vi "main.vi"() -> ()   [LabVIEW 2013, in "Octoplus_LIDAR.lvlib"]
uses:
  <userlib>/Octoplus_LIDAR/Octoplus_LIDAR.lvlib
  <vilib>/Analysis/NI_AALBase.lvlib
panel:
  in  "Nbr of lines in Image":u32=600
  in  "File Path":path=path "D:/Sat25"
  in  "Capture":bool
  in  "Record data":bool
  in  "Timeslot (cw, ts1, ts2)":i32(knob)=1 scale=0.0..2.0
  out "Background":dbl[](graph)
  in  "start":bool
  out "Signal":dbl[][](graph)
  out "iteration":i32
  in  "stop":bool
  in  "error in (no error)":errorcluster
  out "error out":errorcluster
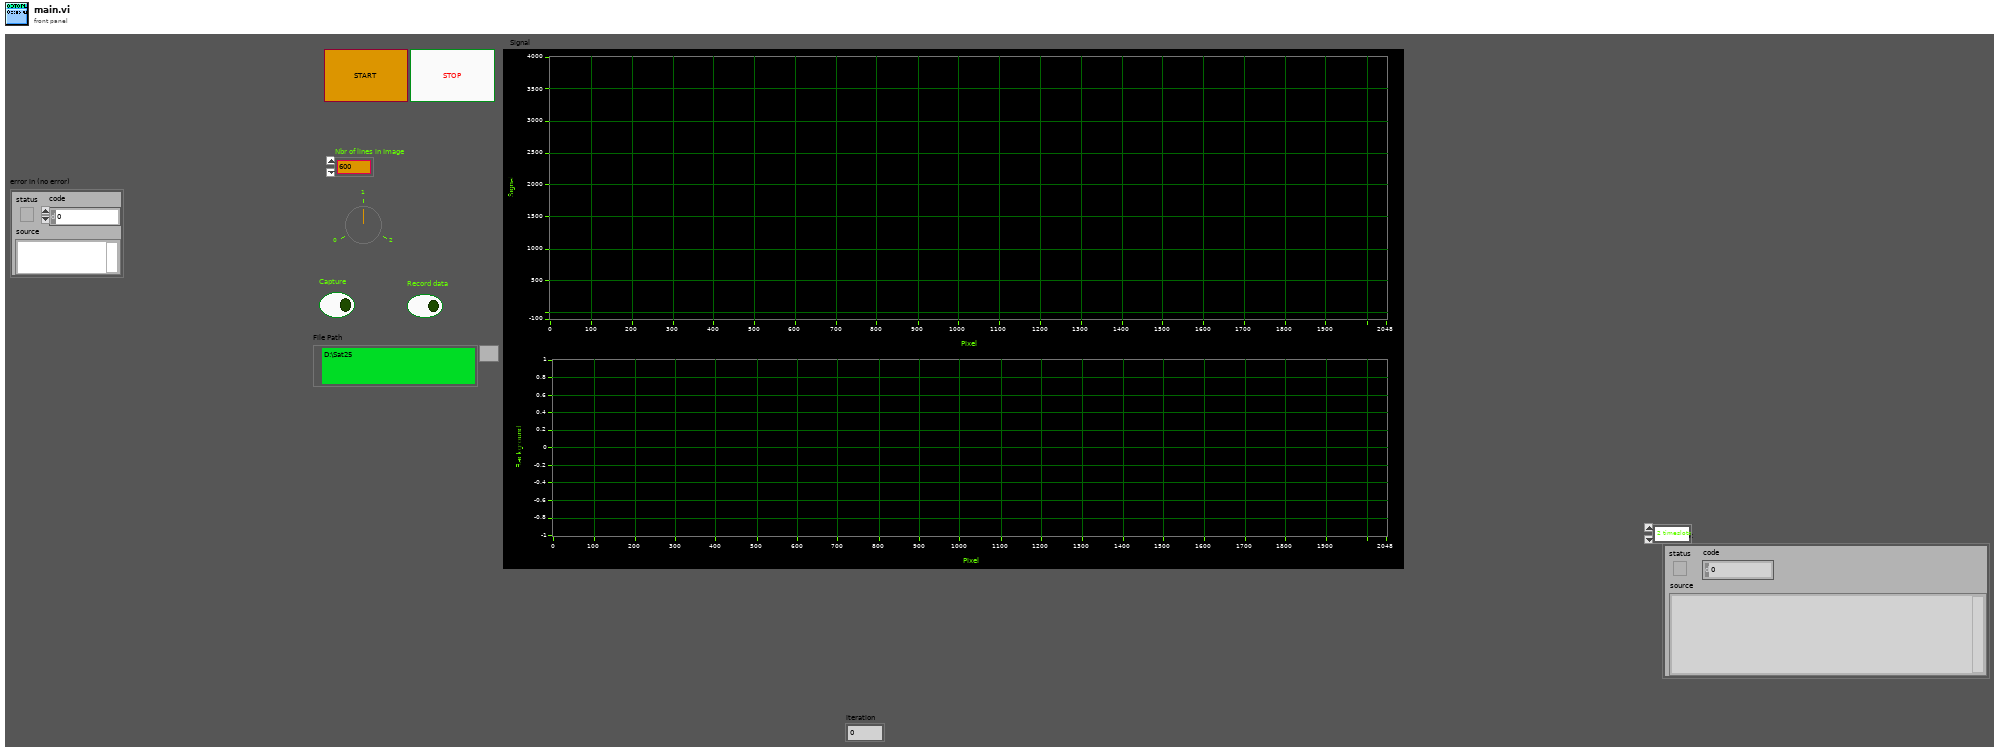
[diagram p1: front panel]
types:
  T1 = cluster{"pcID[0]":i8, "pcID[1]":i8, "pcID[2]":i8, "pcID[3]":i8, "pcID[4]":i8, "pcID[5]":i8, "pcID[6]":i8, "pcID[7]":i8, "pcID[8]":i8, "pcID[9]":i8, "pcID[10]":i8, "pcID[11]":i8, "pcID[12]":i8, "pcID[13]":i8, "pcID[14]":i8, "pcID[15]":i8, "pcID[16]":i8, "pcID[17]":i8, "pcID[18]":i8, "pcID[19]":i8, "pcID[20]":i8, "pcID[21]":i8, "pcID[22]":i8, "pcID[23]":i8, "pcID[24]":i8, "pcID[25]":i8, "pcID[26]":i8, "pcID[27]":i8, "pcID[28]":i8, "pcID[29]":i8, "pcID[30]":i8, "pcID[31]":i8, "pcID[32]":i8, "pcID[33]":i8, "pcID[34]":i8, "pcID[35]":i8, "pcID[36]":i8, "pcID[37]":i8, "pcID[38]":i8, "pcID[39]":i8, "pcID[40]":i8, "pcID[41]":i8, "pcID[42]":i8, "pcID[43]":i8, "pcID[44]":i8, "pcID[45]":i8, "pcID[46]":i8, "pcID[47]":i8, "pcID[48]":i8, "pcID[49]":i8, "pcID[50]":i8, "pcID[51]":i8, "pcID[52]":i8, "pcID[53]":i8, "pcID[54]":i8, "pcID[55]":i8, "pcID[56]":i8, "pcID[57]":i8, "pcID[58]":i8, "pcID[59]":i8, "pcID[60]":i8, "pcID[61]":i8, "pcID[62]":i8, "pcID[63]":i8, "pcID[64]":i8, "pcID[65]":i8, "pcID[66]":i8, "pcID[67]":i8, "pcID[68]":i8, "pcID[69]":i8, "pcID[70]":i8, "pcID[71]":i8, "pcID[72]":i8, "pcID[73]":i8, "pcID[74]":i8, "pcID[75]":i8, "pcID[76]":i8, "pcID[77]":i8, "pcID[78]":i8, "pcID[79]":i8, "pcID[80]":i8, "pcID[81]":i8, "pcID[82]":i8, "pcID[83]":i8, "pcID[84]":i8, "pcID[85]":i8, "pcID[86]":i8, "pcID[87]":i8, "pcID[88]":i8, "pcID[89]":i8, "pcID[90]":i8, "pcID[91]":i8, "pcID[92]":i8, "pcID[93]":i8, "pcID[94]":i8, "pcID[95]":i8, "pcID[96]":i8, "pcID[97]":i8, "pcID[98]":i8, "pcID[99]":i8, "pcID[100]":i8, "pcID[101]":i8, "pcID[102]":i8, "pcID[103]":i8, "pcID[104]":i8, "pcID[105]":i8, "pcID[106]":i8, "pcID[107]":i8, "pcID[108]":i8, "pcID[109]":i8, "pcID[110]":i8, "pcID[111]":i8, "pcID[112]":i8, "pcID[113]":i8, "pcID[114]":i8, "pcID[115]":i8, "pcID[116]":i8, "pcID[117]":i8, "pcID[118]":i8, "pcID[119]":i8, "pcID[120]":i8, "pcID[121]":i8, "pcID[122]":i8, "pcID[123]":i8, "pcID[124]":i8, "pcID[125]":i8, "pcID[126]":i8, "pcID[127]":i8, "pcID[128]":i8, "pcID[129]":i8, "pcID[130]":i8, "pcID[131]":i8, "pcID[132]":i8, "pcID[133]":i8, "pcID[134]":i8, "pcID[135]":i8, "pcID[136]":i8, "pcID[137]":i8, "pcID[138]":i8, "pcID[139]":i8, "pcID[140]":i8, "pcID[141]":i8, "pcID[142]":i8, "pcID[143]":i8, "pcID[144]":i8, "pcID[145]":i8, "pcID[146]":i8, "pcID[147]":i8, "pcID[148]":i8, "pcID[149]":i8, "pcID[150]":i8, "pcID[151]":i8, "pcID[152]":i8, "pcID[153]":i8, "pcID[154]":i8, "pcID[155]":i8, "pcID[156]":i8, "pcID[157]":i8, "pcID[158]":i8, "pcID[159]":i8, "pcID[160]":i8, "pcID[161]":i8, "pcID[162]":i8, "pcID[163]":i8, "pcID[164]":i8, "pcID[165]":i8, "pcID[166]":i8, "pcID[167]":i8, "pcID[168]":i8, "pcID[169]":i8, "pcID[170]":i8, "pcID[171]":i8, "pcID[172]":i8, "pcID[173]":i8, "pcID[174]":i8, "pcID[175]":i8, "pcID[176]":i8, "pcID[177]":i8, "pcID[178]":i8, "pcID[179]":i8, "pcID[180]":i8, "pcID[181]":i8, "pcID[182]":i8, "pcID[183]":i8, "pcID[184]":i8, "pcID[185]":i8, "pcID[186]":i8, "pcID[187]":i8, "pcID[188]":i8, "pcID[189]":i8, "pcID[190]":i8, "pcID[191]":i8, "pcID[192]":i8, "pcID[193]":i8, "pcID[194]":i8, "pcID[195]":i8, "pcID[196]":i8, "pcID[197]":i8, "pcID[198]":i8, "pcID[199]":i8, "pcID[200]":i8, "pcID[201]":i8, "pcID[202]":i8, "pcID[203]":i8, "pcID[204]":i8, "pcID[205]":i8, "pcID[206]":i8, "pcID[207]":i8, "pcID[208]":i8, "pcID[209]":i8, "pcID[210]":i8, "pcID[211]":i8, "pcID[212]":i8, "pcID[213]":i8, "pcID[214]":i8, "pcID[215]":i8, "pcID[216]":i8, "pcID[217]":i8, "pcID[218]":i8, "pcID[219]":i8, "pcID[220]":i8, "pcID[221]":i8, "pcID[222]":i8, "pcID[223]":i8, "pcID[224]":i8, "pcID[225]":i8, "pcID[226]":i8, "pcID[227]":i8, "pcID[228]":i8, "pcID[229]":i8, "pcID[230]":i8, "pcID[231]":i8, "pcID[232]":i8, "pcID[233]":i8, "pcID[234]":i8, "pcID[235]":i8, "pcID[236]":i8, "pcID[237]":i8, "pcID[238]":i8, "pcID[239]":i8, "pcID[240]":i8, "pcID[241]":i8, "pcID[242]":i8, "pcID[243]":i8, "pcID[244]":i8, "pcID[245]":i8, "pcID[246]":i8, "pcID[247]":i8, "pcID[248]":i8, "pcID[249]":i8, "pcID[250]":i8, "pcID[251]":i8, "pcID[252]":i8, "pcID[253]":i8, "pcID[254]":i8, "pcID[255]":i8, "pcID[256]":i8, "pcID[257]":i8, "pcID[258]":i8, "pcID[259]":i8}
  T2 = enum16{"open", "replace", "create", "open or create", "replace or create", "replace or create with confirmation"}
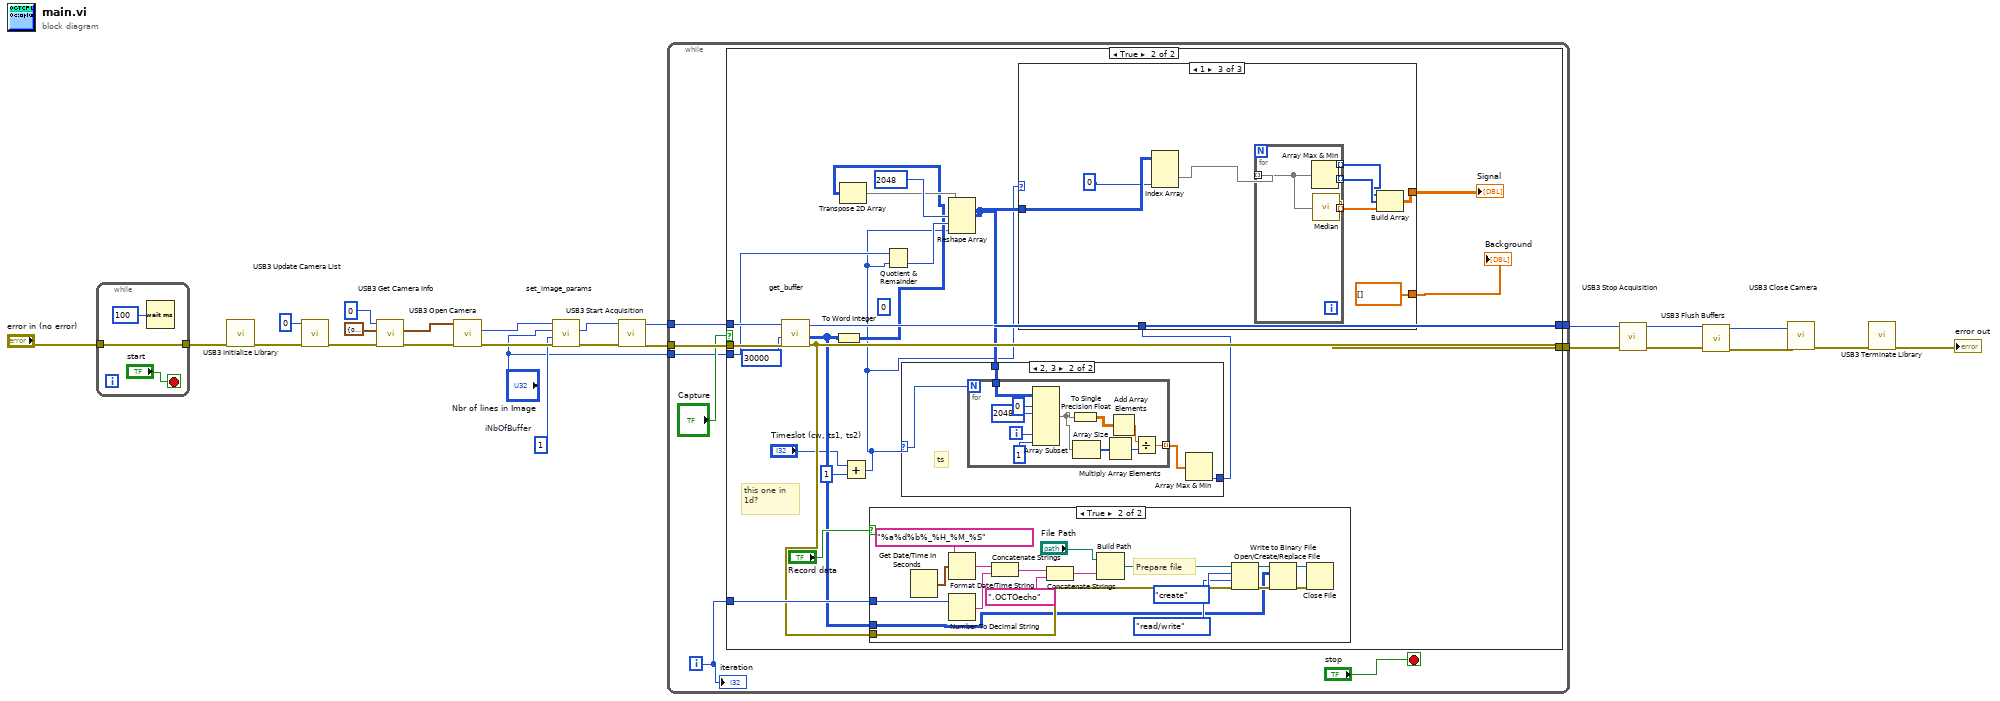
[diagram p0: block diagram]
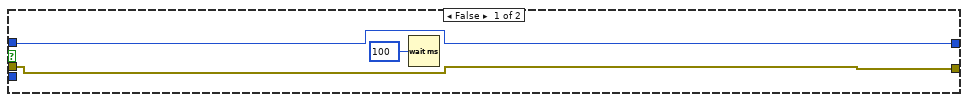
[diagram p2: hidden frame]
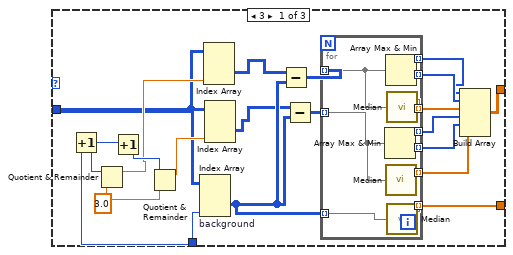
[diagram p3: hidden frame]
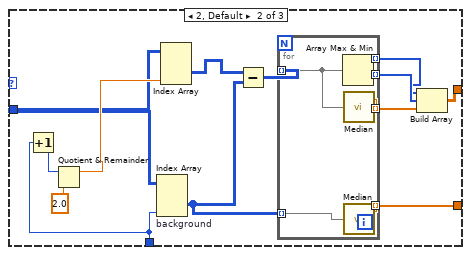
[diagram p4: hidden frame]
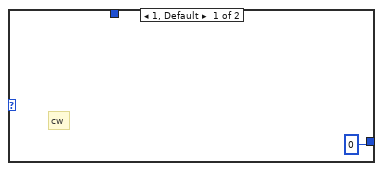
[diagram p6: hidden frame]
diagram:
  w17 = u32 1  # iNbOfBuffer
  n1 = while {
    tunnel: "error in (no error)" -> [w28]
    tunnel: [w28] -> w2
    stop <- "start" stop-if-true
    n2 = Wait (ms)(milliseconds to wait=u32 100) -> ()  [unwired: 1 out]
  }
  n3 = call <userlib>:"USB3 Initialize Library.vi"("error in (no error)"=w2) -> ("error out"=w4:errorcluster)  [unwired: 8 in, 1 out]
  n4 = call <userlib>:"USB3 Update Camera List.vi"("error in (no error)"=w4, "pulNbCameras"=u32 0) -> ("error out"=w22:errorcluster)  [unwired: 7 in, 2 out]
  n5 = call <userlib>:"USB3 Get Camera Info.vi"("error in (no error)"=w22, "pCameraInfo"=T1 {"pcID[0]"=0, "pcID[1]"=0, "pcID[2]"=0, "pcID[3]"=0, "pcID[4]"=0, "pcID[5]"=0, "pcID[6]"=0, "pcID[7]"=0, "pcID[8]"=0, "pcID[9]"=0, "pcID[10]"=0, "pcID[11]"=0, "pcID[12]"=0, "pcID[13]"=0, "pcID[14]"=0, "pcID[15]"=0, "pcID[16]"=0, "pcID[17]"=0, "pcID[18]"=0, "pcID[19]"=0, "pcID[20]"=0, "pcID[21]"=0, "pcID[22]"=0, "pcID[23]"=0, "pcID[24]"=0, "pcID[25]"=0, "pcID[26]"=0, "pcID[27]"=0, "pcID[28]"=0, "pcID[29]"=0, "pcID[30]"=0, "pcID[31]"=0, "pcID[32]"=0, "pcID[33]"=0, "pcID[34]"=0, "pcID[35]"=0, "pcID[36]"=0, "pcID[37]"=0, "pcID[38]"=0, "pcID[39]"=0, "pcID[40]"=0, "pcID[41]"=0, "pcID[42]"=0, "pcID[43]"=0, "pcID[44]"=0, "pcID[45]"=0, "pcID[46]"=0, "pcID[47]"=0, "pcID[48]"=0, "pcID[49]"=0, "pcID[50]"=0, "pcID[51]"=0, "pcID[52]"=0, "pcID[53]"=0, "pcID[54]"=0, "pcID[55]"=0, "pcID[56]"=0, "pcID[57]"=0, "pcID[58]"=0, "pcID[59]"=0, "pcID[60]"=0, "pcID[61]"=0, "pcID[62]"=0, "pcID[63]"=0, "pcID[64]"=0, "pcID[65]"=0, "pcID[66]"=0, "pcID[67]"=0, "pcID[68]"=0, "pcID[69]"=0, "pcID[70]"=0, "pcID[71]"=0, "pcID[72]"=0, "pcID[73]"=0, "pcID[74]"=0, "pcID[75]"=0, "pcID[76]"=0, "pcID[77]"=0, "pcID[78]"=0, "pcID[79]"=0, "pcID[80]"=0, "pcID[81]"=0, "pcID[82]"=0, "pcID[83]"=0, "pcID[84]"=0, "pcID[85]"=0, "pcID[86]"=0, "pcID[87]"=0, "pcID[88]"=0, "pcID[89]"=0, "pcID[90]"=0, "pcID[91]"=0, "pcID[92]"=0, "pcID[93]"=0, "pcID[94]"=0, "pcID[95]"=0, "pcID[96]"=0, "pcID[97]"=0, "pcID[98]"=0, "pcID[99]"=0, "pcID[100]"=0, "pcID[101]"=0, "pcID[102]"=0, "pcID[103]"=0, "pcID[104]"=0, "pcID[105]"=0, "pcID[106]"=0, "pcID[107]"=0, "pcID[108]"=0, "pcID[109]"=0, "pcID[110]"=0, "pcID[111]"=0, "pcID[112]"=0, "pcID[113]"=0, "pcID[114]"=0, "pcID[115]"=0, "pcID[116]"=0, "pcID[117]"=0, "pcID[118]"=0, "pcID[119]"=0, "pcID[120]"=0, "pcID[121]"=0, "pcID[122]"=0, "pcID[123]"=0, "pcID[124]"=0, "pcID[125]"=0, "pcID[126]"=0, "pcID[127]"=0, "pcID[128]"=0, "pcID[129]"=0, "pcID[130]"=0, "pcID[131]"=0, "pcID[132]"=0, "pcID[133]"=0, "pcID[134]"=0, "pcID[135]"=0, "pcID[136]"=0, "pcID[137]"=0, "pcID[138]"=0, "pcID[139]"=0, "pcID[140]"=0, "pcID[141]"=0, "pcID[142]"=0, "pcID[143]"=0, "pcID[144]"=0, "pcID[145]"=0, "pcID[146]"=0, "pcID[147]"=0, "pcID[148]"=0, "pcID[149]"=0, "pcID[150]"=0, "pcID[151]"=0, "pcID[152]"=0, "pcID[153]"=0, "pcID[154]"=0, "pcID[155]"=0, "pcID[156]"=0, "pcID[157]"=0, "pcID[158]"=0, "pcID[159]"=0, "pcID[160]"=0, "pcID[161]"=0, "pcID[162]"=0, "pcID[163]"=0, "pcID[164]"=0, "pcID[165]"=0, "pcID[166]"=0, "pcID[167]"=0, "pcID[168]"=0, "pcID[169]"=0, "pcID[170]"=0, "pcID[171]"=0, "pcID[172]"=0, "pcID[173]"=0, "pcID[174]"=0, "pcID[175]"=0, "pcID[176]"=0, "pcID[177]"=0, "pcID[178]"=0, "pcID[179]"=0, "pcID[180]"=0, "pcID[181]"=0, "pcID[182]"=0, "pcID[183]"=0, "pcID[184]"=0, "pcID[185]"=0, "pcID[186]"=0, "pcID[187]"=0, "pcID[188]"=0, "pcID[189]"=0, "pcID[190]"=0, "pcID[191]"=0, "pcID[192]"=0, "pcID[193]"=0, "pcID[194]"=0, "pcID[195]"=0, "pcID[196]"=0, "pcID[197]"=0, "pcID[198]"=0, "pcID[199]"=0, "pcID[200]"=0, "pcID[201]"=0, "pcID[202]"=0, "pcID[203]"=0, "pcID[204]"=0, "pcID[205]"=0, "pcID[206]"=0, "pcID[207]"=0, "pcID[208]"=0, "pcID[209]"=0, "pcID[210]"=0, "pcID[211]"=0, "pcID[212]"=0, "pcID[213]"=0, "pcID[214]"=0, "pcID[215]"=0, "pcID[216]"=0, "pcID[217]"=0, "pcID[218]"=0, "pcID[219]"=0, "pcID[220]"=0, "pcID[221]"=0, "pcID[222]"=0, "pcID[223]"=0, "pcID[224]"=0, "pcID[225]"=0, "pcID[226]"=0, "pcID[227]"=0, "pcID[228]"=0, "pcID[229]"=0, "pcID[230]"=0, "pcID[231]"=0, "pcID[232]"=0, "pcID[233]"=0, "pcID[234]"=0, "pcID[235]"=0, "pcID[236]"=0, "pcID[237]"=0, "pcID[238]"=0, "pcID[239]"=0, "pcID[240]"=0, "pcID[241]"=0, "pcID[242]"=0, "pcID[243]"=0, "pcID[244]"=0, "pcID[245]"=0, "pcID[246]"=0, "pcID[247]"=0, "pcID[248]"=0, "pcID[249]"=0, "pcID[250]"=0, "pcID[251]"=0, "pcID[252]"=0, "pcID[253]"=0, "pcID[254]"=0, "pcID[255]"=0, "pcID[256]"=0, "pcID[257]"=0, "pcID[258]"=0, "pcID[259]"=0}, "ulIndex"=u32 0) -> ("error out"=w20:errorcluster, "pCameraInfo out"=w21:T1)  [unwired: 6 in, 1 out]
  n6 = call <userlib>:"USB3 Open Camera.vi"("error in (no error)"=w20, "pCameraInfo"=w21) -> ("error out"=w19:errorcluster, "hCamera"=w18:u64)  [unwired: 7 in, 1 out]
  n7 = call <userlib>:"set_image_params.vi"("error in (no error)"=w19, "iNbOfBuffer"=w17, "iImageHeight"="Nbr of lines in Image", "hCamera"=w18) -> ("error out"=w16:errorcluster, "hCamera"=w7:u64)  [unwired: 5 in, 1 out]
  n8 = call <userlib>:"USB3 Start Acquisition.vi"("error in (no error)"=w16, "hCamera"=w7) -> ("error out"=w14:errorcluster, "hCamera"=w15:u64)  [unwired: 7 in, 1 out]
  n9 = while {
    tunnel: w15 -> [w36]
    tunnel: w14 -> [w35]
    tunnel: [w32] -> w13
    tunnel: [w34] -> w10
    tunnel: "Nbr of lines in Image" -> [w30]
    i -> [w29]
    stop <- "stop" stop-if-true
    n10 = case shown="True" "Capture" {
      tunnel: w36 -> [w37 w59]
      tunnel: w35 -> [w38 w58]
      tunnel: [w37 w57] -> w34
      tunnel: [w38 w48] -> w32
      tunnel: w30 -> [_ w53]
      tunnel: w29 -> [_ w49]
      frame False {
        n11 = Wait (ms)(milliseconds to wait=u32 100) -> ()  [unwired: 1 out]
      }
      frame True {
        (unwired) 0 ("index")
        # "this one in\n1d?"
        n12 = call <userlib>:"get_buffer.vi"("error in (no error)"=w58, "ulTimeoutInMs"=u32 30000 ("Buffer timesout (ms)"), "hCamera"=w59) -> ("error out"=w48:errorcluster, "output array"=w43:u16[][], "hCamera out"=w57:u64)  [unwired: 5 in, 1 out]
        n13 = To Word Integer(number=w43) -> (16bit integer=w44:i16[][])
        n14 = Transpose 2D Array(2D array=w44) -> (transposed array=w45:i16[][])
        n15 = Add(x="Timeslot (cw, ts1, ts2)", y=1) -> (x+y=w40:i32)
        n16 = case shown="True" "Record data" {
          tunnel: w48 -> [_ w131]
          tunnel: w43 -> [_ w125]
          tunnel: w49 -> [_ w121]
          frame False {
          }
          frame True {
            # "Prepare file"
            n17 = Get Date/Time In Seconds() -> (seconds since 1Jan1904=w129:timestamp)
            n18 = Format Date/Time String(time format string (%c)="%a%d%b%_%H_%M_%S", seconds (now)=w129) -> (date/time string=w123:string)  [unwired: 1 in]
            n19 = Number To Decimal String(number=w121) -> (decimal integer string=w122:string)  [unwired: 1 in]
            n20 = Concatenate Strings(w123, w122) -> (w124:string)
            n21 = Concatenate Strings(w124, ".OCTOecho") -> (w127:string)
            n22 = Build Path(base path="File Path", name or relative path=w127) -> (appended path=w130:path)
            n23 = Open/Create/Replace File(file path (use dialog)=w130, error in=w131, operation (0:open)=T2."create", access (0:read/write)=enum16{"read/write", "read-only", "write-only"}."read/write") -> (refnum out=w136:refnum<file>, error out=w132:errorcluster)  [unwired: 3 out]
            n24 = Write to Binary File(file (use dialog)=w136, data=w125, error in=w132) -> (refnum out=w134:refnum<file>, error out=w133:errorcluster)  [unwired: 1 in, 3 out]
            n25 = Close File(refnum=w134, error in=w133) -> ()  [unwired: 2 out]
          }
        }
        n26 = Quotient & Remainder(x=w53, y=w40) -> (floor(x/y)=w52:u32)  [unwired: 1 out]
        n27 = Reshape Array(w45, 2048 ("dimension size"), w52, w40) -> (w46:i16[][][])
        n28 = case shown="2, 3" w40 {
          selector: w40 -> [_ w140]
          tunnel: [0 w142] -> w47
          tunnel: w46 -> [_ w141]
          frame 1, Default {
            # "cw"
          }
          frame 2, 3 {
            # "ts"
            n29 = for {
              N: w140 -> [_]
              tunnel: [w153] -> w143 mode=indexing
              tunnel: w141 -> [w148]
              i -> [w150]
              n30 = Array Subset(array=w148, index (dim 0)=0 ("index"), length (dim 0)=2048 ("length"), index (dim 2)=w150, length (dim 2)=1 ("intervals")) -> (w145:i16[][][])  [unwired: 2 in]
              n31 = To Single Precision Float(number=w145) -> (single precision float=w144:sgl[][][])
              n32 = Array Size(array=w145) -> (size(s)=w151:i32[])
              n33 = Multiply Array Elements(1:w151) -> (0:w154:i32)
              n34 = Add Array Elements(numeric array=w144) -> (sum=w152:sgl)
              n35 = Divide(x=w152, y=w154) -> (x/y=w153:sgl)
            }
            n36 = Array Max & Min(array=w143) -> (min index (indices)=w142:i32)  [unwired: 3 out]
          }
        }
        n37 = case shown="1" w40 {
          tunnel: [w77 w100 dbl[] []] -> w55
          tunnel: [w76 w99 w114] -> w51
          tunnel: w47 -> [w71 w95 _]
          tunnel: w46 -> [w68 w93 w112]
          frame 3 {
            w73 = 3.0 ("y")
            n38 = Increment(x=w71) -> (x+1=w74:i32)
            n39 = Quotient & Remainder(x=w74, y=w73) -> (x-y*floor(x/y)=w70:dbl)  [unwired: 1 out]
            n40 = Increment(x=w74) -> (x+1=w72:i32)
            n41 = Quotient & Remainder(x=w72, y=w73) -> (x-y*floor(x/y)=w69:dbl)  [unwired: 1 out]
            n42 = Index Array "background"(array=w68, index (dim 2)=w71) -> (element=w67:i16[][])  [unwired: 2 in]
            n43 = Index Array(array=w68, index (dim 2)=w70) -> (element=w63:i16[][])  [unwired: 2 in]
            n44 = Index Array(array=w68, index (dim 2)=w69) -> (element=w66:i16[][])  [unwired: 2 in]
            n45 = Subtract(x=w63, y=w67) -> (x-y=w65:i16[][])
            n46 = Subtract(x=w66, y=w67) -> (x-y=w64:i16[][])
            n47 = for {
              tunnel: [w89] -> w75 mode=indexing
              tunnel: [w88] -> w79 mode=indexing
              tunnel: [w87] -> w78 mode=indexing
              tunnel: [w86] -> w77 mode=indexing
              tunnel: w67 -> [w85] mode=indexing
              tunnel: w65 -> [w84] mode=indexing
              tunnel: w64 -> [w83] mode=indexing
              tunnel: [w82] -> w62 mode=indexing
              tunnel: [w81] -> w61 mode=indexing
              tunnel: [w80] -> w60 mode=indexing
              n48 = Array Max & Min(array=w83) -> (max value=w82:i16, min value=w81:i16)  [unwired: 2 out]
              n49 = Array Max & Min(array=w84) -> (max value=w87:i16, min value=w88:i16)  [unwired: 2 out]
              n50 = call <vilib>:"Median.vi"("X"=w83) -> ("median"=w80:dbl)  [unwired: 1 out]
              n51 = call <vilib>:"Median.vi"("X"=w84) -> ("median"=w89:dbl)  [unwired: 1 out]
              n52 = call <vilib>:"Median.vi"("X"=w85) -> ("median"=w86:dbl)  [unwired: 1 out]
            }
            n53 = Build Array(w78, w79, w75, w62, w61, w60) -> (w76:dbl[][])
          }
          frame 2, Default {
            n54 = Increment(x=w95) -> (x+1=w97:i32)
            n55 = Quotient & Remainder(x=w97, y=2.0) -> (x-y*floor(x/y)=w94:dbl)  [unwired: 1 out]
            n56 = Index Array "background"(array=w93, index (dim 2)=w95) -> (element=w92:i16[][])  [unwired: 2 in]
            n57 = Index Array(array=w93, index (dim 2)=w94) -> (element=w90:i16[][])  [unwired: 2 in]
            n58 = Subtract(x=w90, y=w92) -> (x-y=w91:i16[][])
            n59 = for {
              tunnel: [w108] -> w98 mode=indexing
              tunnel: [w107] -> w102 mode=indexing
              tunnel: [w106] -> w101 mode=indexing
              tunnel: [w105] -> w100 mode=indexing
              tunnel: w92 -> [w104] mode=indexing
              tunnel: w91 -> [w103] mode=indexing
              n60 = Array Max & Min(array=w103) -> (max value=w106:i16, min value=w107:i16)  [unwired: 2 out]
              n61 = call <vilib>:"Median.vi"("X"=w103) -> ("median"=w108:dbl)  [unwired: 1 out]
              n62 = call <vilib>:"Median.vi"("X"=w104) -> ("median"=w105:dbl)  [unwired: 1 out]
            }
            n63 = Build Array(w101, w102, w98) -> (w99:dbl[][])
          }
          frame 1 {
            n64 = Index Array(array=w112, index (dim 2)=0 ("index (col)")) -> (element=w110:i16[][])  [unwired: 2 in]
            n65 = for {
              tunnel: [w120] -> w113 mode=indexing
              tunnel: [w119] -> w116 mode=indexing
              tunnel: [w118] -> w115 mode=indexing
              tunnel: w110 -> [w117] mode=indexing
              n66 = Array Max & Min(array=w117) -> (max value=w118:i16, min value=w119:i16)  [unwired: 2 out]
              n67 = call <vilib>:"Median.vi"("X"=w117) -> ("median"=w120:dbl)  [unwired: 1 out]
            }
            n68 = Build Array(w115, w116, w113) -> (w114:dbl[][])
          }
        }
        "Signal" <- w51
        "Background" <- w55
      }
    }
    "iteration" <- w29
  }
  n69 = call <userlib>:"USB3 Stop Acquisition.vi"("error in (no error)"=w13, "hCamera"=w10) -> ("error out"=w12:errorcluster, "hCamera out"=w9:u64)  [unwired: 7 in, 1 out]
  n70 = call <userlib>:"USB3 Flush Buffers.vi"("error in (no error)"=w12, "hCamera"=w9) -> ("error out"=w11:errorcluster, "hCamera out"=w8:u64)  [unwired: 7 in, 1 out]
  n71 = call <userlib>:"USB3 Close Camera.vi"("error in (no error)"=w11, "hCamera"=w8) -> ("error out"=w6:errorcluster)  [unwired: 7 in, 2 out]
  n72 = call <userlib>:"USB3 Terminate Library.vi"("error in (no error)"=w6) -> ("error out"=→"error out":errorcluster)  [unwired: 9 in, 1 out]
